vi "ConfigCan.vi"(8 "错误输入（无错误）":errorcluster, 10 "配置波特率":T2={"ABaudrateKbps"=500.0, "AListenOnly"=enum."Normal", "Int120Ohm"=enum."Enable", "EnableChannel"=enum."Enable", "AAppChannel"=0, "硬件类型"=8, "AHwChannel"=0} {"AHwChannel" items=["CHN1", "CHN2", "CHN3", "CHN4", "CHN5", "CHN6", "CHN7", "CHN8", "CHN9", "CHN10", "CHN11", "CHN12", "CHN13", "CHN14", "CHN15", "CHN16", "CHN17", "CHN18", "CHN19", "CHN20", "CHN21", "CHN22", "CHN23", "CHN24", "CHN25", "CHN26", "CHN27", "CHN28", "CHN29", "CHN30", "CHN31", "CHN32", "CHN82"]; "硬件类型" items=["BUS_UNKNOWN_TYPE", "TS_TCP_DEVICE", "XL_USB_DEVICE", "TS_USB_DEVICE", "PEAK_USB_DEVICE", "KVASER_USB_DEVICE", "ZLG_USB_DEVICE", "ICS_USB_DEVICE", "TS_TC1005_DEVICE"]; "AAppChannel" items=["CHN1", "CHN2", "CHN3", "CHN4", "CHN5", "CHN6", "CHN7", "CHN8", "CHN9", "CHN10", "CHN11", "CHN12", "CHN13", "CHN14", "CHN15", "CHN16", "CHN17", "CHN18", "CHN19", "CHN20", "CHN21", "CHN22", "CHN23", "CHN24", "CHN25", "CHN26", "CHN27", "CHN28", "CHN29", "CHN30", "CHN31", "CHN32"]}, 11 "CAN_CardProperties":T1={"应用程序名"="APP", "CAN使用通道数"=1, "LIN使用通道数"=0} {"LIN使用通道数" max=5; "CAN使用通道数" min=1 max=1 step=1}) -> (0 "错误输出":errorcluster, 3 "AAppChannel":i32)   [LabVIEW 2016]
uses:
  CAN_Info.ctl
  CAN_BaudInfo.ctl
panel:
  in  "配置波特率":T2={"ABaudrateKbps"=500.0, "AListenOnly"=enum."Normal", "Int120Ohm"=enum."Enable", "EnableChannel"=enum."Enable", "AAppChannel"=0, "硬件类型"=8, "AHwChannel"=0} {"AHwChannel" items=["CHN1", "CHN2", "CHN3", "CHN4", "CHN5", "CHN6", "CHN7", "CHN8", "CHN9", "CHN10", "CHN11", "CHN12", "CHN13", "CHN14", "CHN15", "CHN16", "CHN17", "CHN18", "CHN19", "CHN20", "CHN21", "CHN22", "CHN23", "CHN24", "CHN25", "CHN26", "CHN27", "CHN28", "CHN29", "CHN30", "CHN31", "CHN32", "CHN82"]; "硬件类型" items=["BUS_UNKNOWN_TYPE", "TS_TCP_DEVICE", "XL_USB_DEVICE", "TS_USB_DEVICE", "PEAK_USB_DEVICE", "KVASER_USB_DEVICE", "ZLG_USB_DEVICE", "ICS_USB_DEVICE", "TS_TC1005_DEVICE"]; "AAppChannel" items=["CHN1", "CHN2", "CHN3", "CHN4", "CHN5", "CHN6", "CHN7", "CHN8", "CHN9", "CHN10", "CHN11", "CHN12", "CHN13", "CHN14", "CHN15", "CHN16", "CHN17", "CHN18", "CHN19", "CHN20", "CHN21", "CHN22", "CHN23", "CHN24", "CHN25", "CHN26", "CHN27", "CHN28", "CHN29", "CHN30", "CHN31", "CHN32"]}
  in  "CAN_CardProperties":T1={"应用程序名"="APP", "CAN使用通道数"=1, "LIN使用通道数"=0} {"LIN使用通道数" max=5; "CAN使用通道数" min=1 max=1 step=1}
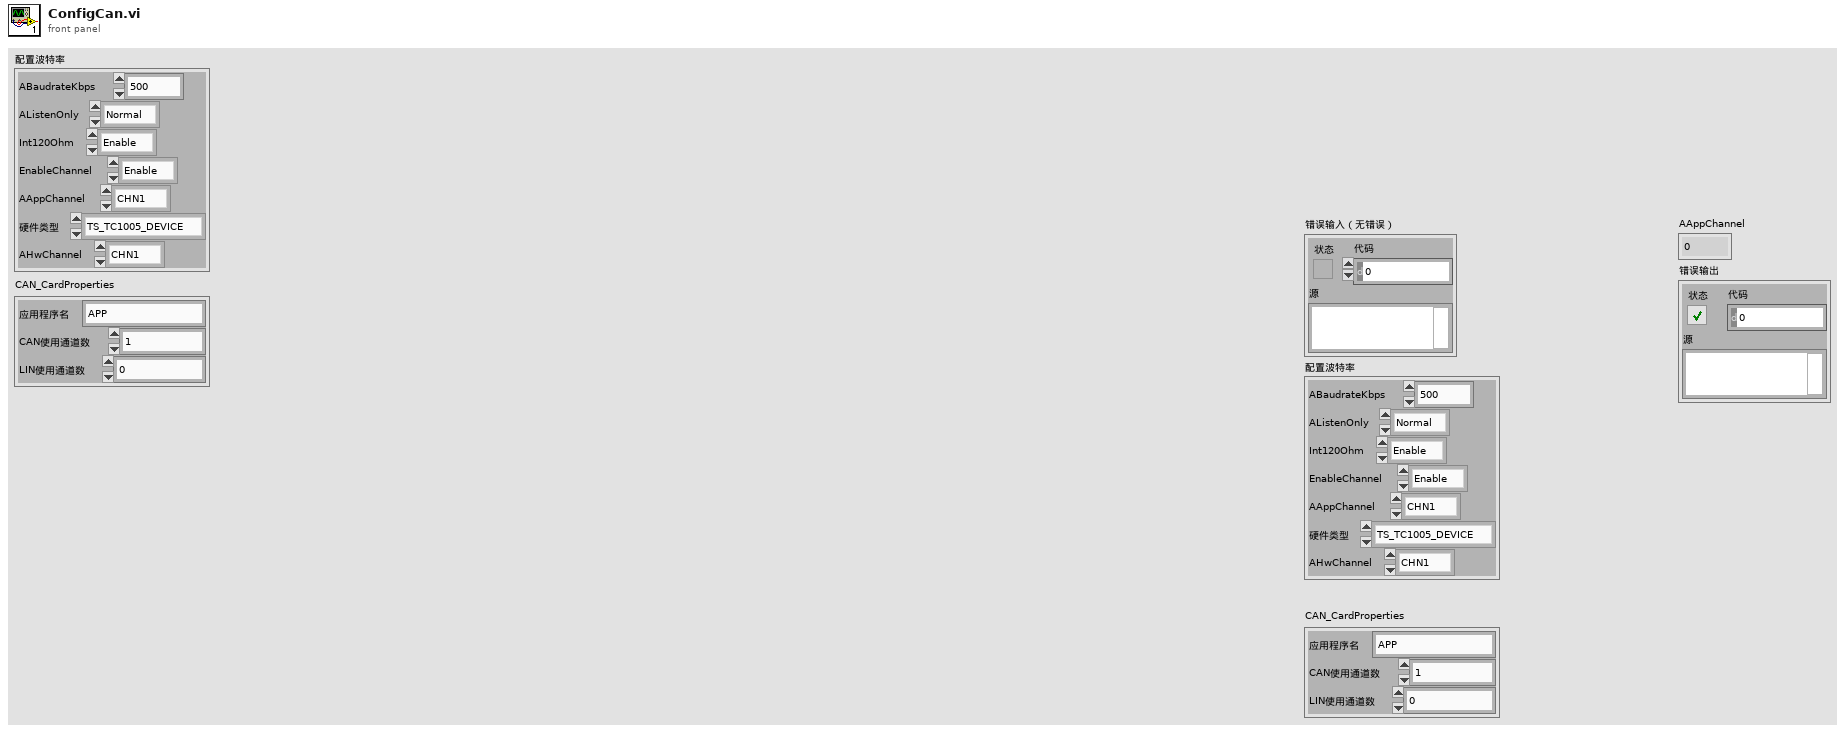
[diagram p1: front panel]
types:
  T1 = typedef "CAN_Info.ctl" = cluster{"应用程序名":string, "CAN使用通道数":u8, "LIN使用通道数":u8}
  T2 = typedef "CAN_BaudInfo.ctl" = cluster{"ABaudrateKbps":sgl, "AListenOnly":enum16{"Normal", "ListenOnly"}, "Int120Ohm":enum16{"Disable", "Enable"}, "EnableChannel":enum16{"Disable", "Enable"}, "AAppChannel":i32, "硬件类型":i32, "AHwChannel":i32}
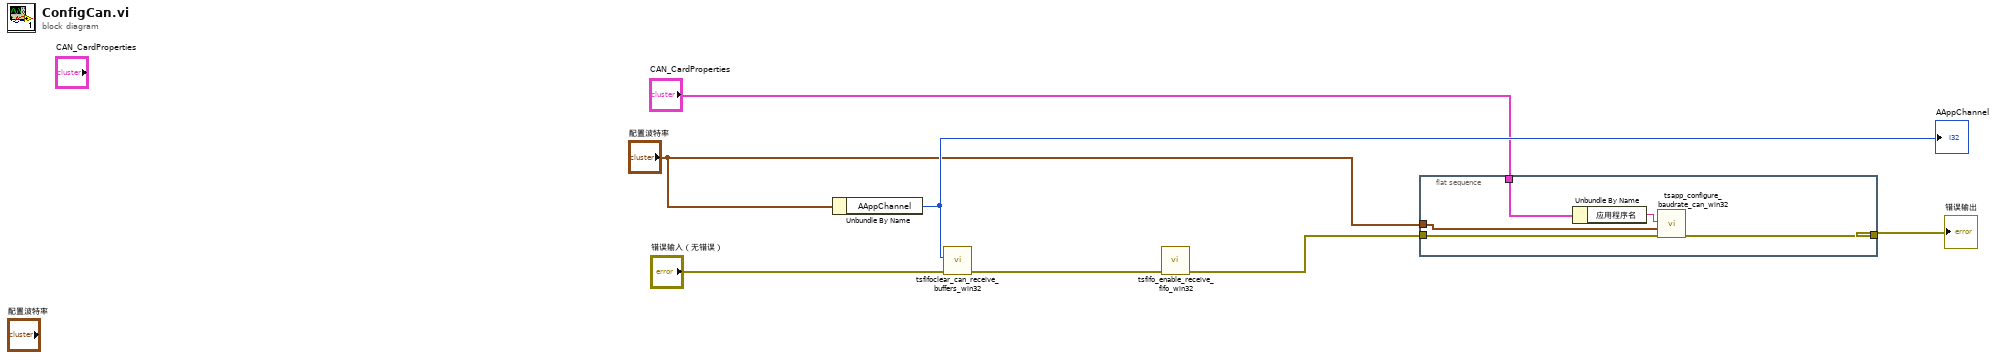
[diagram p0: block diagram]
diagram:
  n1 = Unbundle By Name("配置波特率") -> ("AAppChannel"=w5:i32)
  "AAppChannel" <- w5
  n2 = call "tsfifoclear_can_receive_buffers_win32.vi"("错误输入（无错误）"="错误输入（无错误）", "AAppChannel"=w5) -> ("错误输出"=w7:errorcluster)  [unwired: 8 in, 1 out]
  n3 = call "tsfifo_enable_receive_fifo_win32.vi"("错误输入（无错误）"=w7) -> ("错误输出"=w6:errorcluster)  [unwired: 10 in]
  n4 = flat-sequence {
    tunnel: w6 -> [w12]
    tunnel: "配置波特率" -> [w9]
    tunnel: [w11] -> w2
    tunnel: "CAN_CardProperties" -> [w8]
    frame #0 {
      n5 = Unbundle By Name(w8) -> ("应用程序名"=w10:string)
      n6 = call "tsapp_configure_baudrate_can_win32.vi"("AppName"=w10, "配置波特率"=w9, "错误输入（无错误）"=w12) -> ("错误输出"=w11:errorcluster)  [unwired: 6 in, 1 out]
    }
  }
  "错误输出" <- w2
